vi "Check_Measurement_Setups.vi"(0 "Measurement Setup String":string) -> (1 "Measurement Setup String Out":string, 2 "Error Comments":string)   [LabVIEW 2021]
uses:
  File/Setup_Filetype.ctl
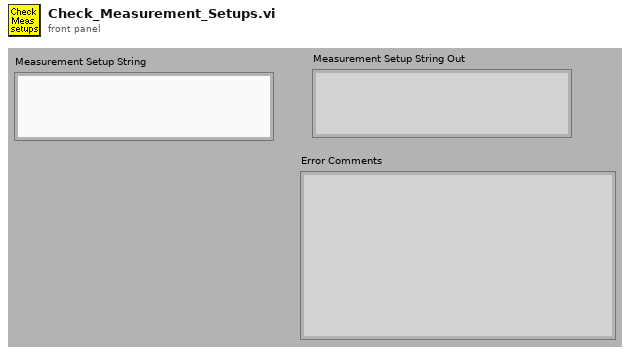
[diagram p1: front panel]
types:
  T1 = typedef "Setup_Filetype.ctl" = enum16{"Measurement Setups", "Calibration Setups", "General", "Results File Plotter Setups", "Speed Calib Tweaks"}
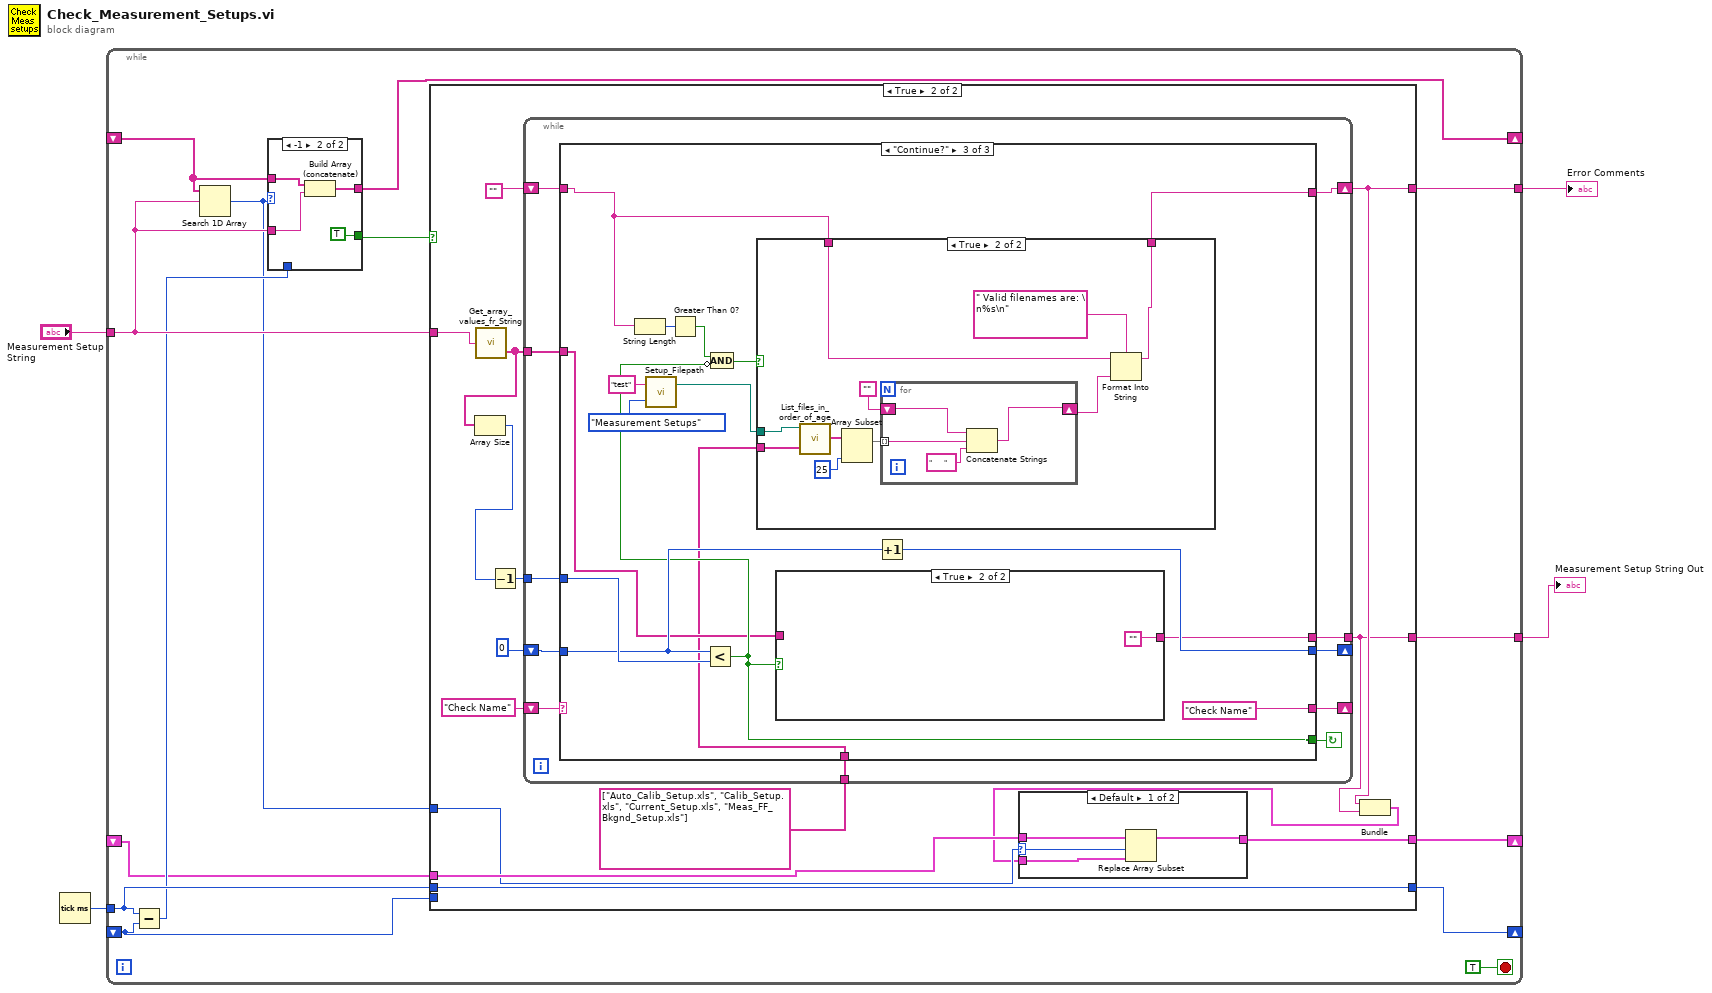
[diagram p0: block diagram]
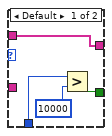
[diagram p2: hidden frame]
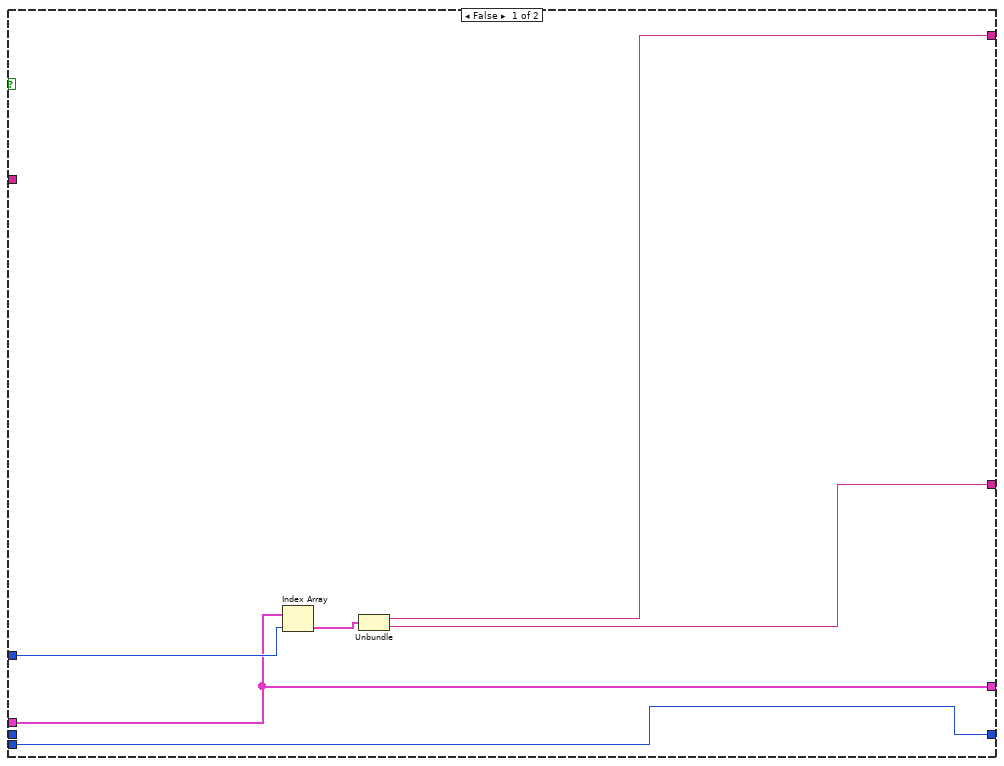
[diagram p3: hidden frame]
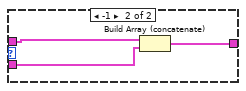
[diagram p4: hidden frame]
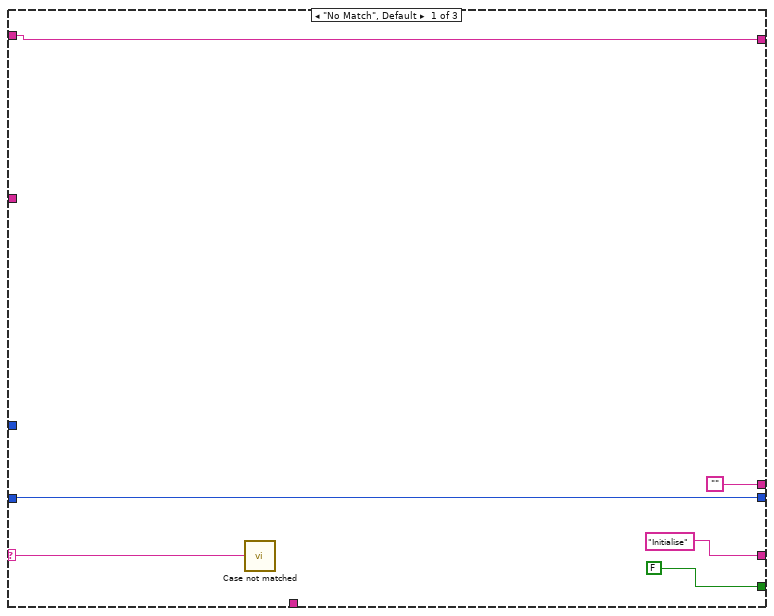
[diagram p5: hidden frame]
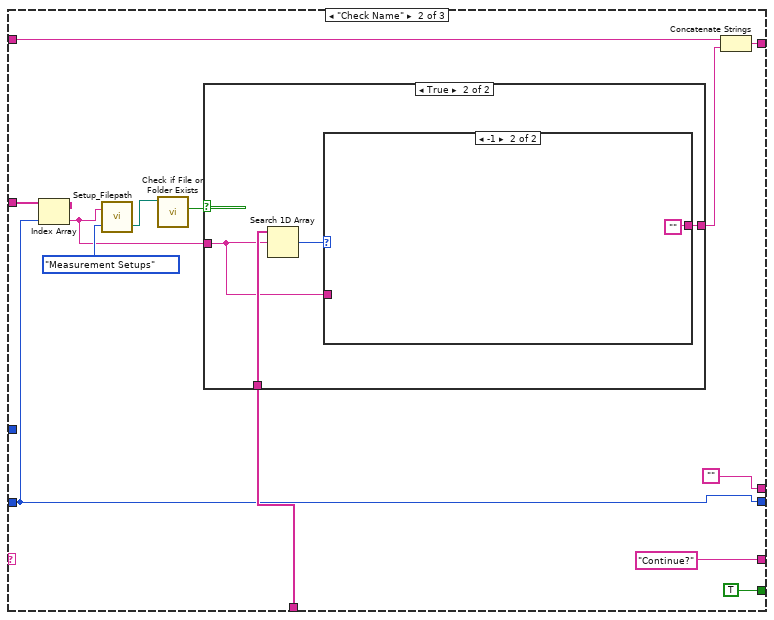
[diagram p6: hidden frame]
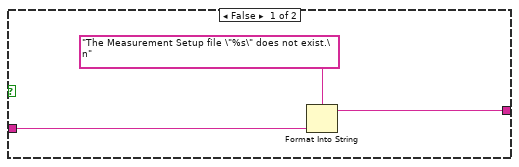
[diagram p7: hidden frame]
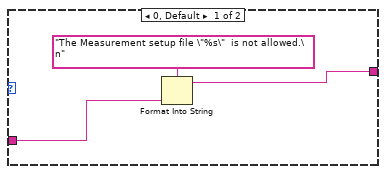
[diagram p8: hidden frame]
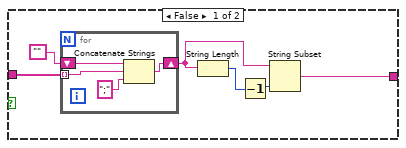
[diagram p9: hidden frame]
diagram:
  n1 = Tick Count (ms)() -> (millisecond timer value=w2:u32)
  n2 = while {
    tunnel: "Measurement Setup String" -> [w16]
    tunnel: [w11] -> w3
    shift-right: [w17] -> _
    shift-left: _ -> [w18]
    shift-right: [w15] -> _
    shift-left: _ -> [w7]
    tunnel: w2 -> [w14]
    shift-right: [w10] -> _
    shift-left: _ -> [w9]
    tunnel: [w5] -> w1
    stop <- TRUE stop-if-true
    n3 = Subtract(x=w14, y=w7) -> (x-y=w13:u32)
    n4 = Search 1D Array(1D array=w18, element=w16) -> (index of element=w8:i32)  [unwired: 1 out]
    n5 = case shown="-1" w8 {
      tunnel: w18 -> [w22 w26]
      tunnel: w16 -> [_ w25]
      tunnel: [w22 w24] -> w17
      tunnel: [w20 TRUE] -> w12
      tunnel: w13 -> [w21 _]
      frame Default {
        n6 = Greater?(x=w21, y=u32 10000) -> (0:w20:bool)
      }
      frame -1 {
        n7 = Build Array (concatenate)(w26, w25) -> (w24:string[])
      }
    }
    n8 = case shown="True" w12 {
      tunnel: w16 -> [_ w45]
      tunnel: [w28 w35] -> w11
      tunnel: [w31 w39] -> w15
      tunnel: w14 -> [_ w39]
      tunnel: [w30 w38] -> w10
      tunnel: w9 -> [w30 w37]
      tunnel: w8 -> [w32 w36]
      tunnel: w7 -> [w31 _]
      tunnel: [w27 w34] -> w5
      frame False {
        n9 = Index Array(array=w30, index=w32) -> (element=w29:cluster{string, string})
        n10 = Unbundle(w29) -> (w28:string, w27:string)
      }
      frame True {
        n11 = call "Get_array_values_fr_String.vi"("String Value"=w45) -> ("String array"=w44:string[])  [unwired: 1 out]
        n12 = Array Size(array=w44) -> (size(s)=w43:i32)
        n13 = Decrement(x=w43) -> (x-1=w42:i32)
        n14 = while {
          shift-left: "Check Name" -> [w63]
          shift-right: [w64] -> _
          shift-right: [w59] -> _
          shift-left: 0 -> [w62]
          tunnel: w44 -> [w61]
          tunnel: w42 -> [w60]
          shift-right: [w58] -> w35
          shift-left: "" -> [w57]
          tunnel: string[] ["Auto_Calib_Setup.xls", "Calib_Setup.xls", "Current_Setup.xls", "Meas_FF_Bkgnd_Setup.xls"] ("file names") -> [w56]
          tunnel: [w55] -> w34
          stop <- w65 continue-if-true
          n15 = case shown="\"Continue?\"" w63 {
            selector: w63 -> [w67 _ _]
            tunnel: [FALSE TRUE w102] -> w65
            tunnel: ["Initialise" "Continue?" "Check Name"] -> w64
            tunnel: w62 -> [w69 w76 w110]
            tunnel: w61 -> [_ w84 w101]
            tunnel: w60 -> [_ _ w111]
            tunnel: [w69 w76 w109] -> w59
            tunnel: [w68 w82 w103] -> w58
            tunnel: w57 -> [w68 w80 w104]
            tunnel: w56 -> [_ w77 w100]
            tunnel: ["" "" w96] -> w55
            frame "No Match", Default {
              n16 = call "Case not matched.vi"("Case Name not Matched"=w67) -> ()
            }
            frame "Check Name" {
              n17 = Index Array(array=w84, index=w76) -> (element=w74:string)
              n18 = call "Setup_Filepath.vi"("Setup File Type"=Setup_Filetype."Measurement Setups", "Filename in"=w74) -> ("Filename Out"=w73:path)  [unwired: 1 out]
              n19 = call <vilib>:"Check if File or Folder Exists.vi"("path"=w73) -> ("file or folder exists?"=w83:bool)  [unwired: 1 in, 9 out]
              n20 = case shown="True" w83 {
                tunnel: w74 -> [w86 w88]
                tunnel: [w85 w89] -> w81
                tunnel: w77 -> [_ w91]
                frame False {
                  n21 = Format Into String(format string="The Measurement Setup file \"%s\" does not exist.\n" ("Format String"), w86) -> (resulting string=w85:string)  [unwired: 2 in, 1 out]
                }
                frame True {
                  n22 = Search 1D Array(1D array=w91, element=w88) -> (index of element=w90:i32)  [unwired: 1 out]
                  n23 = case shown="-1" w90 {
                    tunnel: [w93 ""] -> w89
                    tunnel: w88 -> [w92 _]
                    frame 0, Default {
                      n24 = Format Into String(format string="The Measurement setup file \"%s\"  is not allowed.\n" ("f"), w92) -> (resulting string=w93:string)  [unwired: 2 in, 1 out]
                    }
                    frame -1 {
                    }
                  }
                }
              }
              n25 = Concatenate Strings(w80, w81) -> (w82:string)
            }
            frame "Continue?" {
              n26 = String Length(string=w104) -> (length=w107:i32)
              n27 = call "Setup_Filepath.vi"("Setup File Type"=Setup_Filetype."Measurement Setups", "Filename in"="test") -> ("Directory"=w98:path)  [unwired: 1 out]
              n28 = Greater Than 0?(x=w107) -> (x > 0?=w106:bool)
              n29 = Less?(x=w110, y=w111) -> (x < y?=w102:bool)
              n30 = Compound Arithmetic op=AND(w106, invert w102) -> (w105:bool)
              n31 = case shown="True" w105 {
                tunnel: w104 -> [w123 w127]
                tunnel: [w123 w126] -> w103
                tunnel: w100 -> [_ w125]
                tunnel: w98 -> [_ w124]
                frame False {
                }
                frame True {
                  n32 = call "List_files_in_order_of_age.vi"("Files to Hide"=w125, "Folder"=w124) -> ("file names"=w129:string[])  [unwired: 9 in]
                  n33 = Array Subset(array=w129, length=25 ("Array Length")) -> (w131:string[])  [unwired: 1 in]
                  n34 = for {
                    shift-right: [w136] -> w133
                    shift-left: "" -> [w137]
                    tunnel: w131 -> [w135] mode=indexing
                    n35 = Concatenate Strings(w137, w135, "      " ("Substring")) -> (w136:string)
                  }
                  n36 = Format Into String(format string=" Valid filenames are: \n%s\n" ("Format String"), initial string=w127, w133) -> (resulting string=w126:string)  [unwired: 1 in, 1 out]
                }
              }
              n37 = case shown="True" w102 {
                tunnel: w101 -> [w117 _]
                tunnel: [w112 ""] -> w96
                frame False {
                  n38 = for {
                    shift-right: [w118] -> w114
                    shift-left: "" -> [w121]
                    tunnel: w117 -> [w120] mode=indexing
                    n39 = Concatenate Strings(w121, w120, ";") -> (w118:string)
                  }
                  n40 = String Length(string=w114) -> (length=w115:i32)
                  n41 = Decrement(x=w115) -> (x-1=w113:i32)
                  n42 = String Subset(string=w114, length (rest)=w113) -> (substring=w112:string)  [unwired: 1 out]
                }
                frame True {
                }
              }
              n43 = Increment(x=w110) -> (x+1=w109:i32)
            }
          }
        }
        n44 = Bundle(w35, w34) -> (w33:cluster{string, string})  [unwired: 1 in]
        n45 = case shown="Default" w36 {
          selector: w36 -> [w49 _]
          tunnel: w33 -> [w50 w54]
          tunnel: w37 -> [w51 w53]
          tunnel: [w48 w52] -> w38
          frame Default {
            n46 = Replace Array Subset(array=w51, new element=w50, index=w49) -> (w48:cluster{string, string}[])
          }
          frame -1 {
            n47 = Build Array (concatenate)(w53, w54) -> (w52:cluster{string, string}[])
          }
        }
      }
    }
  }
  "Error Comments" <- w3
  "Measurement Setup String Out" <- w1
